vi "Handle SET.vi"(8 "error in (no error)":errorcluster, 9 "data":variant, 10 "parameter":string, 11 "Inst.Transport in":refnum<class "Inst.Transport.lvclass">) -> (0 "error out":errorcluster, 2 "data out":variant, 3 "Inst.Transport out":refnum<class "Inst.Transport.lvclass">)   [LabVIEW 2019, in "Inst.Transport.lvclass"]
uses:
  Inst.Transport.lvclass
  <userlib>/LevyLab/Instrument Framework/Instrument Types/SCPI/Instrument.SCPI.lvclass
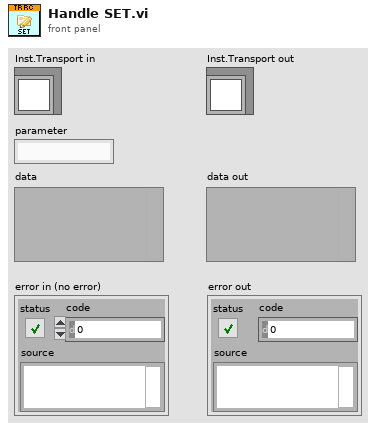
[diagram p1: front panel]
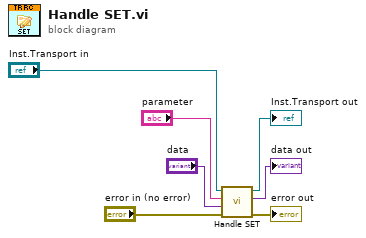
[diagram p0: block diagram]
diagram:
  n1 = call-parent "Handle SET.vi"("error in (no error)"="error in (no error)", "data"="data", "parameter"="parameter", "Instrument in"="Inst.Transport in") -> ("error out"=→"error out":errorcluster, "data out"=→"data out":variant, "Instrument out"=→"Inst.Transport out":refnum<class "Inst.Transport.lvclass">)  [unwired: 5 in]
